vi "Create Frame Pattern Script.vi"(8 "error in (no error)":errorcluster, 9 "ChipID":u8, 10 "Frame_Data":T1={"Pattern_Name"="", "Operation Mode"=enum."Normal", "BurstLength"=enum."0", "FSN"=0, "Start_Addr"=0, "Data"=[], "R/W?"=enum."Read", "Opcode"=[], "ChipID"=1, "num of wait cycle of read"=0} {"Data" format="%x"; "Start_Addr" format="%x"}, 11 "BML_Frame_Command in":refnum<class "BML_Frame_Command.lvclass">) -> (0 "error out":errorcluster, 3 "BML_Frame_Command out":refnum<class "BML_Frame_Command.lvclass">)   [LabVIEW 2018, in "BML_Frame_Command.lvclass"]
uses:
  BML_Frame_Command.lvclass
  C:/P4 Workspace/PC Client/Solutions/5g_eap/HiSi/trunk/1.0/BML_Pattern_Gen_Refactor/Classes/BML_Frame_Root/BML_Frame_Root.lvclass
  Config_Read/Frame_Data.ctl
  Config_Read/OperationMode.ctl
  Config_Read/BurstLength.ctl
  Config_Read/RW_Option.ctl
  BML_Frame_Root/Special Frame.ctl
  BML_Frame_Root/BML_Frame_Root.lvclass/BML_Frame_Root.ctl
  BML_Frame_Root/BML_Frame_Root.lvclass
  Config_Read/Config_Read_BML.lvclass
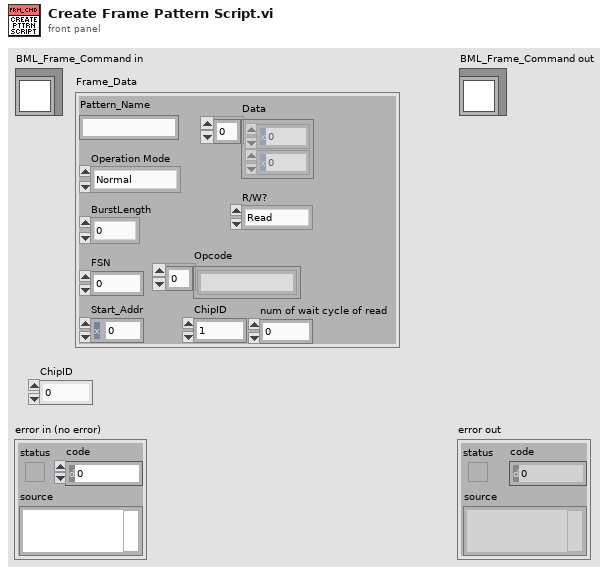
[diagram p1: front panel]
types:
  T1 = typedef "Config_Read_BML.lvclass/Frame_Data.ctl" = cluster{"Pattern_Name":string, "Operation Mode":T2, "BurstLength":T3, "FSN":u8, "Start_Addr":u16, "Data":u8[], "R/W?":T4, "Opcode":string[], "ChipID":u8, "num of wait cycle of read":i8}
  T2 = typedef "Config_Read_BML.lvclass/OperationMode.ctl" = enum8{"Normal", "ImmeEffect", "InitSlaveID", "LoadData"}
  T3 = typedef "Config_Read_BML.lvclass/BurstLength.ctl" = enum8{"0", "2", "3", "4", "5", "8", "16", "32"}
  T4 = typedef "Config_Read_BML.lvclass/RW_Option.ctl" = enum16{"Read", "Write", "R/W"}
  T5 = typedef "BML_Frame_Root.lvclass/Special Frame.ctl" = enum16{"Sync Header", "Protocol Header", "SW Trig", "SetID State", "Out SetID State", "SW Reset", "Wait", "SPI 4W FRM Start", "SPI 4W Wait", "SPI 4W FRM End", "SPI 4W Write Cmd", "SPI RD Collect Cmd", "SPI RD Value Cmd", "SPI 3W FRM Start", "SPI 3W Write Cmd", "SPI 3W FRM End", "SPI 3W Wait", "SPI 3W RD Cmd"}
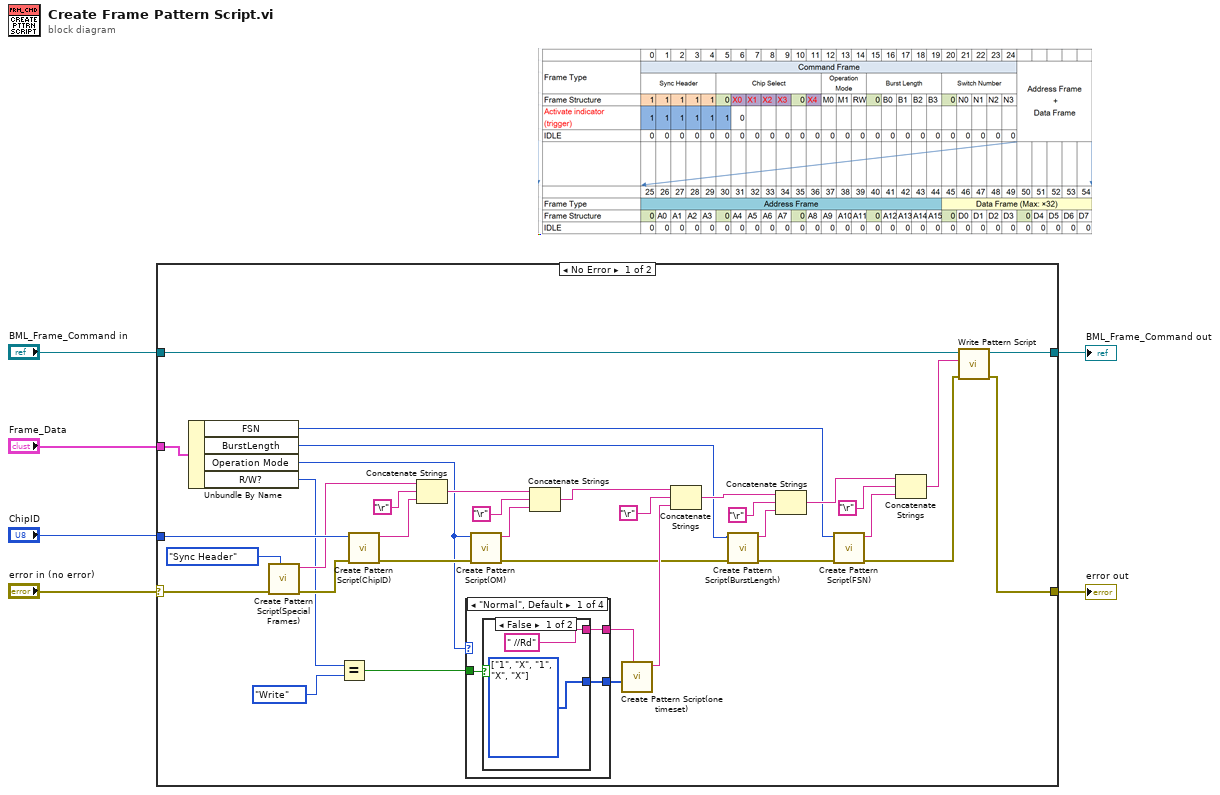
[diagram p0: block diagram]
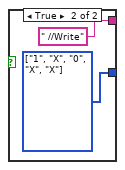
[diagram p2: hidden frame]
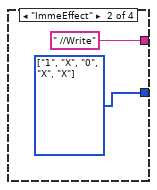
[diagram p3: hidden frame]
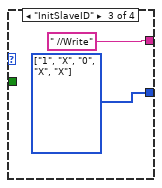
[diagram p4: hidden frame]
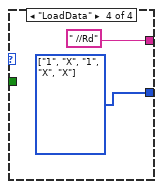
[diagram p5: hidden frame]
diagram:
  n1 = case shown="No Error" "error in (no error)" {
    selector: "error in (no error)" -> [w33 w57]
    tunnel: "BML_Frame_Command in" -> [w17 w56]
    tunnel: [w13 w57] -> w1
    tunnel: [w16 w56] -> w2
    tunnel: "Frame_Data" -> [w42 _]
    tunnel: "ChipID" -> [w34 _]
    frame No Error {
      n2 = Unbundle By Name(w42) -> ("FSN"=w20:u8, "BurstLength"=w22:T3, "Operation Mode"=w12:T2, "R/W?"=w9:T4)
      n3 = call "Create Pattern Script(Special Frames).vi"("Special Frame Type"=Special_Frame."Sync Header", "error in (no error)"=w33) -> ("error out"=w31:errorcluster, "string out"=w30:string)  [unwired: 8 in]
      n4 = Equal?(x=w9, y=RW_Option."Write") -> (x = y?=w7:bool)
      n5 = call "Create Pattern Script(ChipID).vi"("error in (no error)"=w31, "ChipID"=w34) -> ("error out"=w26:errorcluster, "Script out"=w28:string)  [unwired: 8 in]
      n6 = Concatenate Strings(w30, "\r", w28) -> (w27:string)
      n7 = case shown="\"Normal\", Default" w12 {
        tunnel: [w43 w51 w52 w54] -> w11
        tunnel: [w44 " //Write" " //Write" " //Rd"] -> w10
        tunnel: w7 -> [w45 _ _ _]
        frame "Normal", Default {
          n8 = case shown="False" w45 {
            tunnel: [" //Rd" " //Write"] -> w44
            tunnel: [w47 w48] -> w43
            frame False {
              w47 = enum16{"0", "1", "L", "H", "X", "V", "D", "M"}[] [enum."1", enum."X", enum."1", enum."X", enum."X"] items=["0", "1", "L", "H", "X", "V", "D", "M"] ("PinState")
            }
            frame True {
              w48 = enum16{"0", "1", "L", "H", "X", "V", "D", "M"}[] [enum."1", enum."X", enum."0", enum."X", enum."X"] items=["0", "1", "L", "H", "X", "V", "D", "M"] ("PinState")
            }
          }
        }
        frame "ImmeEffect" {
          w51 = enum16{"0", "1", "L", "H", "X", "V", "D", "M"}[] [enum."1", enum."X", enum."0", enum."X", enum."X"] items=["0", "1", "L", "H", "X", "V", "D", "M"] ("PinState")
        }
        frame "InitSlaveID" {
          w52 = enum16{"0", "1", "L", "H", "X", "V", "D", "M"}[] [enum."1", enum."X", enum."0", enum."X", enum."X"] items=["0", "1", "L", "H", "X", "V", "D", "M"] ("PinState")
        }
        frame "LoadData" {
          w54 = enum16{"0", "1", "L", "H", "X", "V", "D", "M"}[] [enum."1", enum."X", enum."1", enum."X", enum."X"] items=["0", "1", "L", "H", "X", "V", "D", "M"] ("PinState")
        }
      }
      n9 = call "Create Pattern Script(OM).vi"("error in (no error)"=w26, "Operation Mode in"=w12) -> ("error out"=w23:errorcluster, "OM string out"=w25:string)  [unwired: 8 in]
      n10 = Concatenate Strings(w27, "\r", w25) -> (w36:string)
      n11 = call "Create Pattern Script(one timeset).vi"("Notes"=w10, "PinState"=w11) -> ("string out"=w24:string)  [unwired: 9 in]
      n12 = Concatenate Strings(w36, "\r", w24) -> (w39:string)
      n13 = call "Create Pattern Script(BurstLength).vi"("error in (no error)"=w23, "BurstLength"=w22) -> ("error out"=w19:errorcluster, "String"=w21:string)  [unwired: 8 in]
      n14 = Concatenate Strings(w39, "\r", w21) -> (w38:string)
      n15 = call "Create Pattern Script(FSN).vi"("error in (no error)"=w19, "FSN"=w20) -> ("error out"=w14:errorcluster, "String"=w18:string)  [unwired: 8 in]
      n16 = Concatenate Strings(w38, "\r", w18) -> (w15:string)
      n17 = call "Write Pattern Script.vi"("error in (no error)"=w14, "Pattern Script"=w15, "BML_Frame_Root in"=w17) -> ("error out"=w13:errorcluster, "BML_Frame_Root out"=w16:refnum<class "BML_Frame_Command.lvclass">)  [unwired: 7 in]
    }
    frame Error {
    }
  }
  "error out" <- w1
  "BML_Frame_Command out" <- w2
